vi "LineMove.vi"(2 "handle in":i32, 3 "Rotate":bool, 4 "ROI":T1, 5 "Pixel Size (nm)":dbl) -> (1 "handle out":i32)   [LabVIEW 2011]
uses:
  MCL libraries/MicroDrive.dll
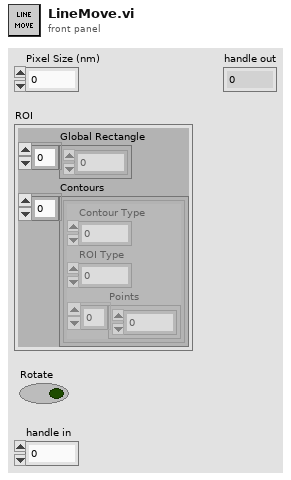
[diagram p1: front panel]
types:
  T1 = cluster{"Global Rectangle":i32[], "Contours":cluster{"Contour Type":u32, "ROI Type":u32, "Points":i32[]}[]}
  T2 = typedef "IMAQ Line" = cluster{"Start X":i32, "Start Y":i32, "End X":i32, "End Y":i32}
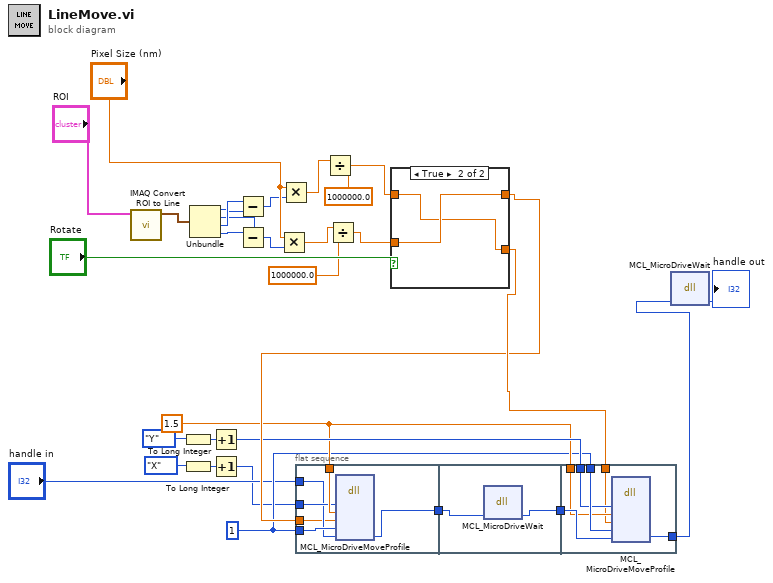
[diagram p0: block diagram]
diagram:
  w13 = 1 ("roundingX")
  w14 = 1.5 ("velocityX")
  n1 = call "IMAQ Convert ROI to Line"("ROI Descriptor"="ROI") -> ("Line"=w23:T2)  [unwired: 8 in, 1 out]
  n2 = To Long Integer(number=enum16{"X", "Y"}."Y" ("Axis 2")) -> (32bit integer=w8:i32)
  n3 = To Long Integer(number=enum16{"X", "Y"}."X" ("Axis 2")) -> (32bit integer=w7:i32)
  n4 = Unbundle(w23) -> ("Start X"=w21:i32, "Start Y"=w19:i32, "End X"=w22:i32, "End Y"=w20:i32)
  n5 = Increment(x=w8) -> (x+1=w15:i32)
  n6 = Increment(x=w7) -> (x+1=w11:i32)
  n7 = Subtract(x=w22, y=w21) -> (x-y=w27:i32)
  n8 = Subtract(x=w20, y=w19) -> (x-y=w28:i32)
  n9 = Multiply(x="Pixel Size (nm)", y=w28) -> (x*y=w3:dbl)
  n10 = Multiply(x="Pixel Size (nm)", y=w27) -> (x*y=w6:dbl)
  n11 = flat-sequence {
    tunnel: w14 -> [w37]
    tunnel: w11 -> [w36]
    tunnel: w13 -> [w35]
    tunnel: "handle in" -> [w34]
    tunnel: [w33] -> w31
    tunnel: w25 -> [w32]
    tunnel: [w38] -> w30
    tunnel: w31 -> [w39]
    tunnel: [w41] -> w16
    tunnel: w30 -> [w45]
    tunnel: w13 -> [w44]
    tunnel: w14 -> [w43]
    tunnel: w15 -> [w42]
    tunnel: w26 -> [w40]
    frame #0 {
      n12 = dll-call lib="F:/Vlad/Labview code/PZM_photogate/MCL libraries/MicroDrive.dll" fn="MCL_MicroDriveMoveProfile" ("MicroDrive.dll:\nMCL_MicroDriveMoveProfile")("axis"=w36, "velocity"=w37, "distance"=w32, "rounding"=w35, "handle"=w34) -> ("handle"=w33:i32)  [unwired: 7 in, 3 out]
    }
    frame #1 {
      n13 = dll-call lib="F:/Vlad/Labview code/PZM_photogate/MCL libraries/MicroDrive.dll" fn="MCL_MicroDriveWait"("handle"=w39) -> ("handle"=w38:i32)  [unwired: 4 in, 2 out]
    }
    frame #2 {
      n14 = dll-call lib="F:/Vlad/Labview code/PZM_photogate/MCL libraries/MicroDrive.dll" fn="MCL_MicroDriveMoveProfile" ("MicroDrive.dll:\nMCL_MicroDriveMoveProfile")("axis"=w42, "velocity"=w43, "distance"=w40, "rounding"=w44, "handle"=w45) -> ("handle"=w41:i32)  [unwired: 7 in, 3 out]
    }
  }
  n15 = Divide(x=w6, y=1000000.0) -> (x/y=w4:dbl)
  n16 = Divide(x=w3, y=1000000.0) -> (x/y=w1:dbl)
  n17 = case shown="True" "Rotate" {
    tunnel: w4 -> [w47 w48]
    tunnel: [w47 w49] -> w25
    tunnel: [w46 w48] -> w26
    tunnel: w1 -> [w46 w49]
    frame False {
    }
    frame True {
    }
  }
  n18 = dll-call lib="F:/Vlad/Labview code/PZM_photogate/MCL libraries/MicroDrive.dll" fn="MCL_MicroDriveWait"("handle"=w16) -> ("handle"=→"handle out":i32)  [unwired: 4 in, 2 out]
